vi "MotionProfiles_Control.vi"(8 "error in (no error)":errorcluster, 9 "PhoenixMotorControlDevRef Slave":T1={"DeviceStatus"={"status"=FALSE, "code"=0, "source"=""}, "Type"=enum."PWM", "PWM"={"PWM Channel"=enum."Invalid", "DeadBand"={"Name"="", "maxPositivePwm"=0, "minPositivePwm"=0, "centerPwm"=0, "maxNegativePwm"=0, "minNegativePwm"=0, "angularRange"=0}}, "CAN"={"Device Number"=0, "SetOutput VI Ref"=variant(refnum<vi> refnum), "GetOutput VI Ref"=variant(refnum<vi> refnum), "Enable VI Ref"=variant(refnum<vi> refnum), "Disable VI Ref"=variant(refnum<vi> refnum), "Data"=variant}, "Invert"=FALSE, "DIO PWM"={"PWM \"Enable\" Channel"=enum."Invalid", "DIOChannel"=enum."Invalid", "PWM Rate"=0.0}}, 11 "MotionProfiles in":refnum<class "MotionProfiles.lvclass">) -> (0 "error out":errorcluster, 3 "MotionProfiles out":refnum<class "MotionProfiles.lvclass">)   [LabVIEW 2018, in "MotionProfiles.lvclass"]
uses:
  MotionProfiles.lvclass
  <vilib>/Rock Robotics/WPI/MotorControl/WPI_MotorControlDeviceRef.ctl
  <vilib>/Rock Robotics/WPI/MotorControl/WPI_MotorControlType.ctl
  <vilib>/Rock Robotics/SystemInterfaces/DIO/FPGA_DIOPWMChannel.ctl
  <vilib>/Rock Robotics/WPI/PWM/WPI_PWMDeadband.ctl
  <vilib>/Rock Robotics/SystemInterfaces/DIO/FPGA_DIOChannel.ctl
  <vilib>/Rock Robotics/WPI/ThirdParty/Phoenix-LabVIEW/Motor Controller/Controls/CTRE_Phoenix_MotorControl_ControlMode.ctl
  MotionProfiles.lvclass/MotionProfiles.ctl
  MotionProfile_TalonSetValueEnum.ctl
  MotionProfile_InternalStateEnum.ctl
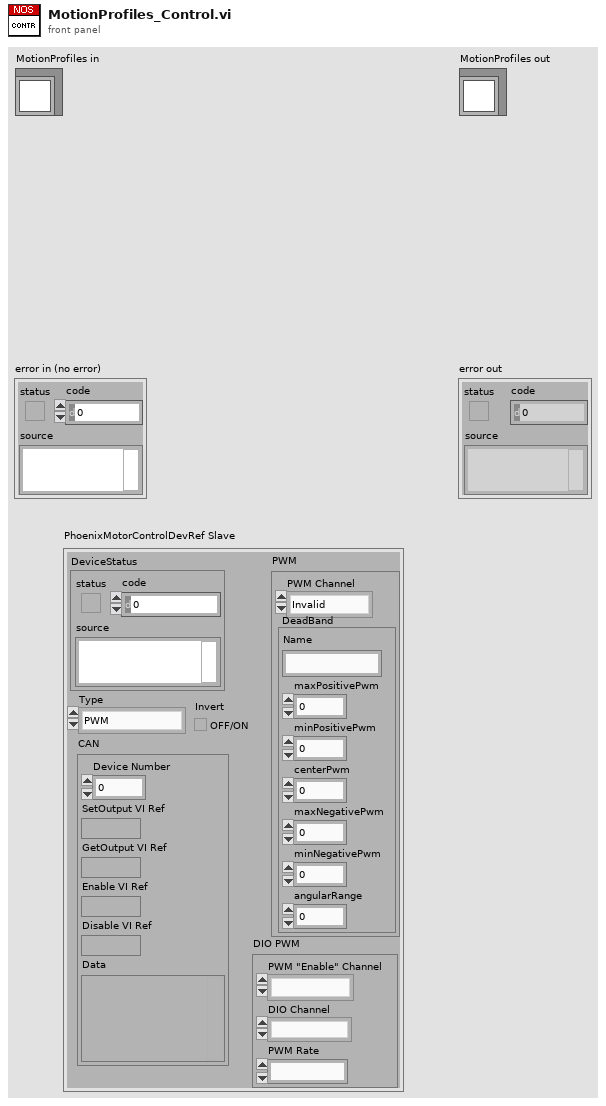
[diagram p1: front panel]
types:
  T1 = typedef "WPI_MotorControlDeviceRef.ctl" = cluster{"DeviceStatus":errorcluster, "Type":T2, "PWM":cluster{"PWM Channel":T3, "DeadBand":T4}, "CAN":cluster{"Device Number":u8, "SetOutput VI Ref":variant, "GetOutput VI Ref":variant, "Enable VI Ref":variant, "Disable VI Ref":variant, "Data":variant}, "Invert":bool, "DIO PWM":cluster{"PWM \"Enable\" Channel":T3, "DIOChannel":T5, "PWM Rate":dbl}}
  T2 = typedef "WPI_MotorControlType.ctl" = enum16{"PWM", "CAN", "DIO PWM"}
  T3 = typedef "FPGA_DIOPWMChannel.ctl" = enum8{"PWM 0", "PWM 1", "PWM 2", "PWM 3", "PWM 4", "PWM 5", "PWM 6", "PWM 7", "PWM 8", "PWM 9", "PWM MXP 0", "PWM MXP 1", "PWM MXP 2", "PWM MXP 3", "PWM MXP 4", "PWM MXP 5", "PWM MXP 6", "PWM MXP 7", "PWM MXP 8", "PWM MXP 9", "Invalid"}
  T4 = typedef "WPI_PWMDeadband.ctl" = cluster{"Name":string, "maxPositivePwm":i32, "minPositivePwm":i32, "centerPwm":i32, "maxNegativePwm":i32, "minNegativePwm":i32, "angularRange":u16}
  T5 = typedef "FPGA_DIOChannel.ctl" = enum8{"DIO 0", "DIO 1", "DIO 2", "DIO 3", "DIO 4", "DIO 5", "DIO 6", "DIO 7", "DIO 8", "DIO 9", "DIO MXP 0", "DIO MXP 1", "DIO MXP 2", "DIO MXP 3", "DIO MXP 4", "DIO MXP 5", "DIO MXP 6", "DIO MXP 7", "DIO MXP 8", "DIO MXP 9", "DIO MXP 10", "DIO MXP 11", "DIO MXP 12", "DIO MXP 13", "DIO MXP 14", "DIO MXP 15", "SPI Port CS1", "SPI Port CS2", "SPI Port CS3", "SPI Port MISO", "SPI Port MOSI", "Invalid"}
  T6 = typedef "MotionProfiles.lvclass/MotionProfile_InternalStateEnum.ctl" = enum16{"Nothing", "Send Points to Talon", "Run Profile"}
  T7 = typedef "MotionProfiles.lvclass/MotionProfile_TalonSetValueEnum.ctl" = enum16{"Disable", "Enable", "Hold"}
  T8 = typedef "CTRE_Phoenix_MotorControl_ControlMode.ctl" = u16
  T9 = cluster{"Top Buffer Remaining":i32, "Top Buffer Count":i32, "Bottom Buffer Count":i32, "Has Underrun?":bool, "Is Underrun?":bool, "Active Point Valid?":bool, "Is Last?":bool, "Profile Slot Select 0":i32, "Output Enable":i32, "Time Duration (ms)":i32, "Profile Slot Select 1":i32}
  T10 = typedef "MotionProfiles.lvclass/MotionProfile_TrajectoryPoint.ctl" = cluster{"Duration (ms)":u8, "Velocity (u/100ms)":dbl, "Position (units)":dbl, "Profile Slot Select":u8, "Is Last":bool, "Velocity Only":bool, "Zero Position":bool, "Compress Code":u8, "Same Velocity":i32, "Delta Position":i32, "Count":u8, "Invert Motors?":bool}
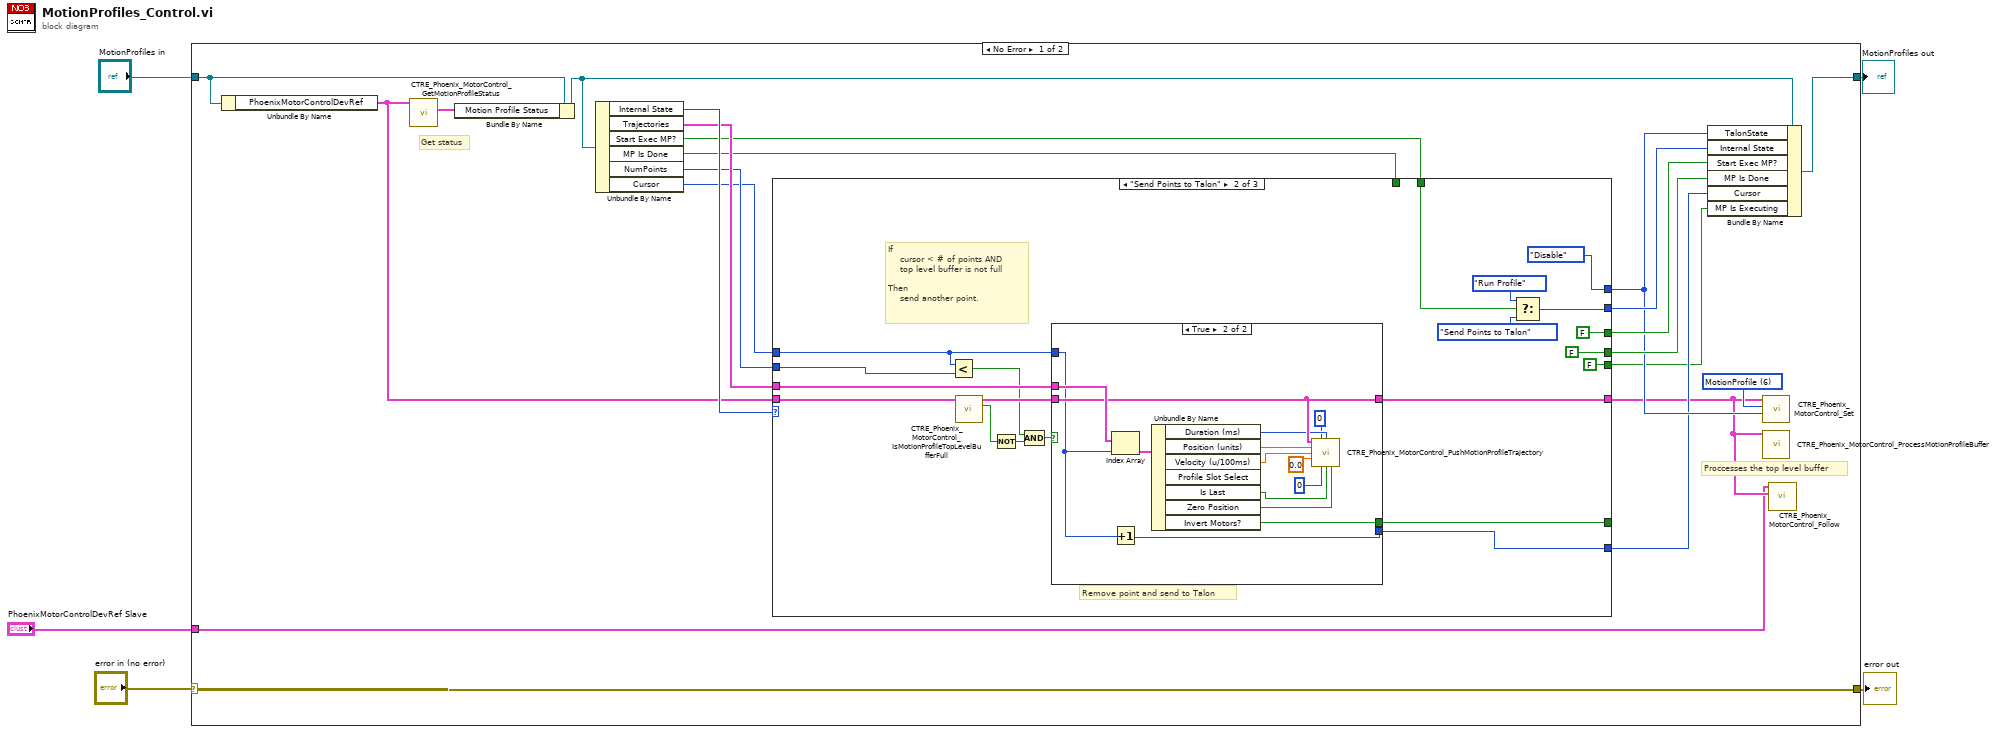
[diagram p0: block diagram]
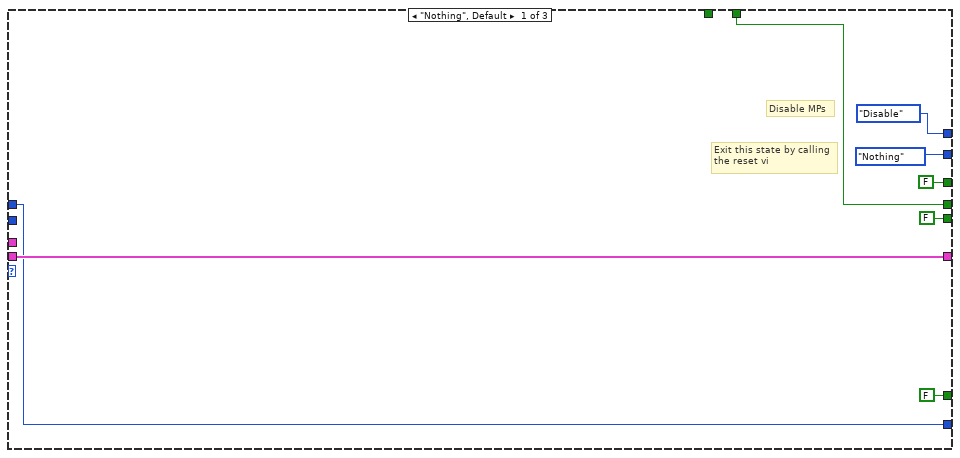
[diagram p2: hidden frame]
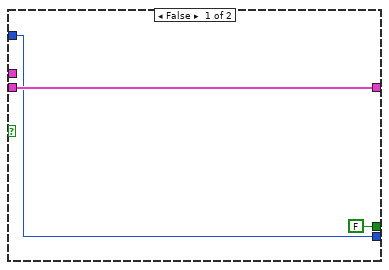
[diagram p3: hidden frame]
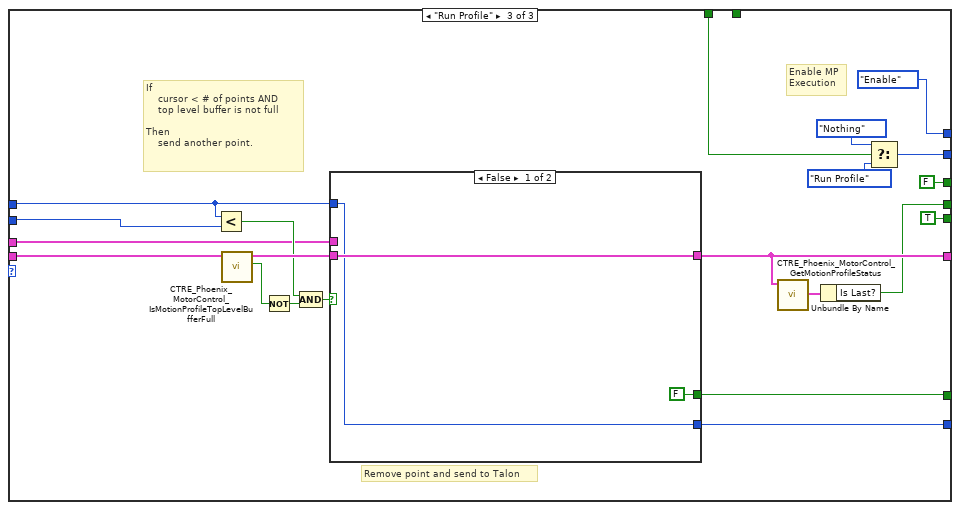
[diagram p4: hidden frame]
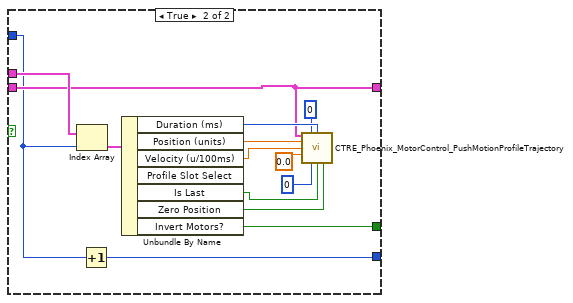
[diagram p5: hidden frame]
diagram:
  n1 = case shown="No Error" "error in (no error)" {
    selector: "error in (no error)" -> [w26 w111]
    tunnel: [w26 w111] -> w4
    tunnel: [w25 w110] -> w2
    tunnel: "MotionProfiles in" -> [w9 w110]
    tunnel: "PhoenixMotorControlDevRef Slave" -> [w6 _]
    frame No Error {
      w17 = T8 6 items=["PercentOutput"=0, "Position"=1, "Velocity"=2, "Current"=3, "Follower"=5, "MotionProfile"=6, "MotionMagic"=7, "MotionMagicArc"=8, "MotionProfileArc"=10, "Disabled"=15] ("Control Mode")
      # "Get status"
      # "Proccesses the top level buffer"
      n2 = Unbundle By Name(w9) -> ("PhoenixMotorControlDevRef"=w11:T1)
      n3 = call <vilib>:"CTRE_Phoenix_MotorControl_GetMotionProfileStatus.vi"("PhoenixMotorControlDevRef"=w11) -> ("Motion Profile Status"=w8:T9)  [unwired: 8 in, 2 out]
      n4 = Bundle By Name(cluster=w9, "Motion Profile Status"=w8) -> (w10:refnum<class "MotionProfiles.lvclass">)
      n5 = Unbundle By Name(w10) -> ("Internal State"=w24:T6, "Trajectories"=w23:T10[], "Start Exec MP?"=w22:bool, "MP Is Done"=w20:bool, "NumPoints"=w19:u32, "Cursor"=w13:u32)
      n6 = case shown="\"Send Points to Talon\"" w24 {
        tunnel: [MotionProfile_InternalStateEnum."Nothing" ("Internal State") w52 w90] -> w16
        tunnel: [MotionProfile_TalonSetValueEnum."Disable" ("TalonSetValue") MotionProfile_TalonSetValueEnum."Disable" ("TalonSetValue") MotionProfile_TalonSetValueEnum."Enable" ("TalonSetValue")] -> w15
        tunnel: w23 -> [_ w51 w79]
        tunnel: w11 -> [w32 w43 w78]
        tunnel: w22 -> [w29 w46 _]
        tunnel: [FALSE ("Start Exec MP?") FALSE ("Start Exec MP?") FALSE] -> w21
        tunnel: w20 -> [_ _ w87]
        tunnel: w19 -> [_ w38 w80]
        tunnel: [w29 FALSE ("Mot Prof Active Is Last") w74] -> w18
        tunnel: [w32 w42 w76] -> w7
        tunnel: [w31 w40 w77] -> w14
        tunnel: w13 -> [w31 w39 w81]
        tunnel: [FALSE FALSE TRUE] -> w12
        tunnel: [FALSE ("Invert Motors?") w35 w72] -> _
        frame "Nothing", Default {
          # "Exit this state by calling\nthe reset vi"
          # "Disable MPs"
        }
        frame "Send Points to Talon" {
          # "If \n    cursor < # of points AND\n    top level buffer is not full\n    \nThen \n    send another point."
          # "Remove point and send to Talon"
          n7 = Less?(x=w39, y=w38) -> (x < y?=w37:bool)
          n8 = call <vilib>:"CTRE_Phoenix_MotorControl_IsMotionProfileTopLevelBufferFull.vi"("PhoenixMotorControlDevRef"=w43) -> ("Is Motion Profile Top Level Buffer Full?"=w44:bool, "PhoenixMotorControlDevRef"=w41:T1)  [unwired: 8 in, 1 out]
          n9 = Not(x=w44) -> (.not. x?=w45:bool)
          n10 = Compound Arithmetic op=AND(w37, w45) -> (w47:bool)
          n11 = case shown="True" w47 {
            tunnel: w51 -> [_ w71]
            tunnel: [w57 w69] -> w42
            tunnel: w41 -> [w57 w69]
            tunnel: [w56 w61] -> w40
            tunnel: w39 -> [w56 w60]
            tunnel: [FALSE ("Invert Motors?") w58] -> w35
            frame False {
            }
            frame True {
              n12 = Index Array(array=w71, index=w60) -> (element=w70:T10)
              n13 = Increment(x=w60) -> (x+1=w61:u32)
              n14 = Unbundle By Name(w70) -> ("Duration (ms)"=w68:u8, "Position (units)"=w66:dbl, "Velocity (u/100ms)"=w65:dbl, "Is Last"=w62:bool, "Zero Position"=w59:bool, "Invert Motors?"=w58:bool)  [unwired: 1 out]
              n15 = call <vilib>:"CTRE_Phoenix_MotorControl_PushMotionProfileTrajectory.vi"("PhoenixMotorControlDevRef"=w69, "profileSlotSelect1"=0, "durationMs"=w68, "position"=w66, "velocity"=w65, "auxiliaryPos"=0.0 ("headingDeg"), "profileSlotSelect0"=0, "isLastPoint?"=w62, "Zero Position?"=w59) -> ()  [unwired: 5 in, 2 out]
            }
          }
          n16 = Select(t=MotionProfile_InternalStateEnum."Run Profile" ("Internal State"), s=w46, f=MotionProfile_InternalStateEnum."Send Points to Talon" ("Internal State")) -> (s? t:f=w52:T6)
        }
        frame "Run Profile" {
          # "If \n    cursor < # of points AND\n    top level buffer is not full\n    \nThen \n    send another point."
          # "Remove point and send to Talon"
          # "Enable MP\nExecution"
          n17 = Less?(x=w81, y=w80) -> (x < y?=w82:bool)
          n18 = call <vilib>:"CTRE_Phoenix_MotorControl_IsMotionProfileTopLevelBufferFull.vi"("PhoenixMotorControlDevRef"=w78) -> ("Is Motion Profile Top Level Buffer Full?"=w84:bool, "PhoenixMotorControlDevRef"=w83:T1)  [unwired: 8 in, 1 out]
          n19 = Not(x=w84) -> (.not. x?=w85:bool)
          n20 = Compound Arithmetic op=AND(w82, w85) -> (w86:bool)
          n21 = case shown="False" w86 {
            tunnel: w79 -> [_ w109]
            tunnel: [w95 w98] -> w76
            tunnel: w83 -> [w95 w98]
            tunnel: [w94 w99] -> w77
            tunnel: w81 -> [w94 w97]
            tunnel: [FALSE ("Invert Motors?") w96] -> w72
            frame False {
            }
            frame True {
              n22 = Index Array(array=w109, index=w97) -> (element=w108:T10)
              n23 = Increment(x=w97) -> (x+1=w99:u32)
              n24 = Unbundle By Name(w108) -> ("Duration (ms)"=w107:u8, "Position (units)"=w105:dbl, "Velocity (u/100ms)"=w104:dbl, "Is Last"=w101:bool, "Zero Position"=w100:bool, "Invert Motors?"=w96:bool)  [unwired: 1 out]
              n25 = call <vilib>:"CTRE_Phoenix_MotorControl_PushMotionProfileTrajectory.vi"("PhoenixMotorControlDevRef"=w98, "profileSlotSelect1"=0, "durationMs"=w107, "position"=w105, "velocity"=w104, "auxiliaryPos"=0.0 ("headingDeg"), "profileSlotSelect0"=0, "isLastPoint?"=w101, "Zero Position?"=w100) -> ()  [unwired: 5 in, 2 out]
            }
          }
          n26 = call <vilib>:"CTRE_Phoenix_MotorControl_GetMotionProfileStatus.vi"("PhoenixMotorControlDevRef"=w76) -> ("Motion Profile Status"=w75:T9)  [unwired: 8 in, 2 out]
          n27 = Unbundle By Name(w75) -> ("Is Last?"=w74:bool)
          n28 = Select(t=MotionProfile_InternalStateEnum."Nothing" ("Internal State"), s=w87, f=MotionProfile_InternalStateEnum."Run Profile" ("Internal State")) -> (s? t:f=w90:T6)
        }
      }
      n29 = Bundle By Name(cluster=w10, "TalonState"=w15, "Internal State"=w16, "Start Exec MP?"=w21, "MP Is Done"=w18, "Cursor"=w14, "MP Is Executing"=w12) -> (w25:refnum<class "MotionProfiles.lvclass">)
      n30 = call <vilib>:"CTRE_Phoenix_MotorControl_Set.vi"("Output"=w15, "Control Mode"=w17, "PhoenixMotorControlDevRef"=w7) -> ()  [unwired: 7 in, 2 out]
      n31 = call <vilib>:"CTRE_Phoenix_MotorControl_ProcessMotionProfileBuffer.vi"("PhoenixMotorControlDevRef"=w7) -> ()  [unwired: 13 in, 2 out]
      n32 = call <vilib>:"CTRE_Phoenix_MotorControl_Follow.vi"("Master Controller to Follow"=w7, "PhoenixMotorControlDevRef"=w6) -> ()  [unwired: 8 in, 2 out]
    }
    frame Error {
    }
  }
  "error out" <- w4
  "MotionProfiles out" <- w2
